vi "Folder Reuse Warning.vi"(8 "error in":errorcluster, 10 "folder names":string[](array[string]), 11 "project ref":refnum<vi>) -> (0 "error out":errorcluster, 3 "proceed?":bool)   [LabVIEW 2021, in "MeasurementClient Editor.lvlib"]
uses:
  MeasurementClient Editor.lvlib
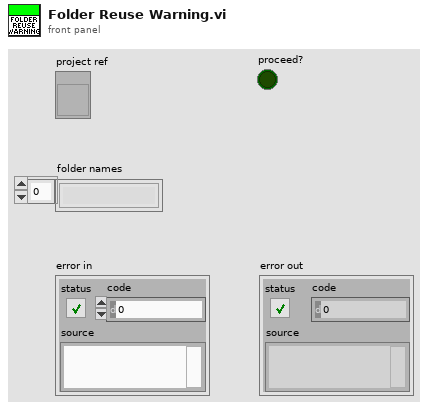
[diagram p1: front panel]
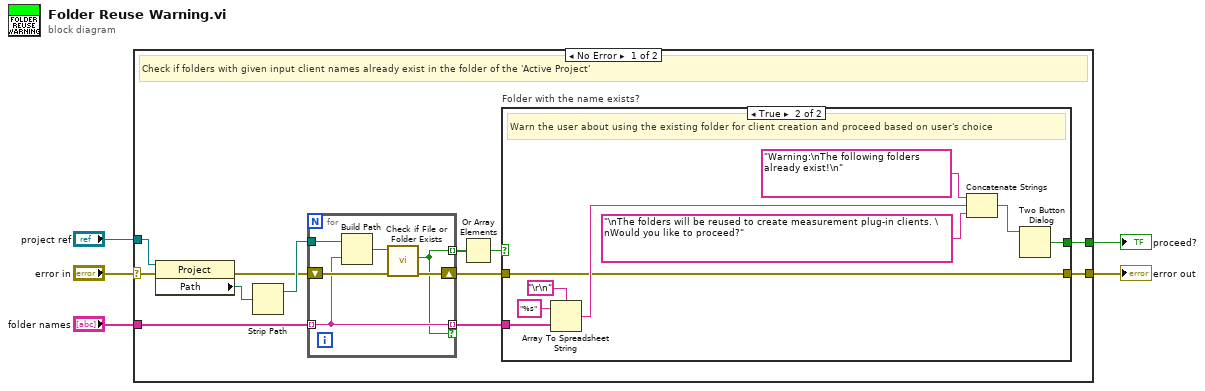
[diagram p0: block diagram]
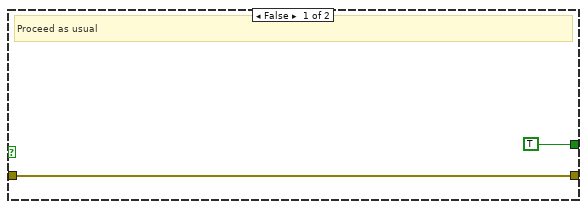
[diagram p2: hidden frame]
diagram:
  n1 = case shown="No Error" "error in" {
    selector: "error in" -> [w17 w35]
    tunnel: [w13 w35] -> w2
    tunnel: "folder names" -> [w12 _]
    tunnel: "project ref" -> [w6 _]
    tunnel: [w9 _] -> w1
    frame No Error {
      # "Check if folders with given input client names already exist in the folder of the 'Active Project'"
      n2 = property class="Project"(reference=w6, error in=w17) -> (error out=w8:errorcluster, "Path"=w16:path)  [unwired: 1 out]
      n3 = Strip Path(path=w16) -> (stripped path=w15:path)  [unwired: 1 out]
      n4 = for {
        tunnel: w15 -> [w34]
        tunnel: w12 -> [w30] mode=indexing
        tunnel: [w29] -> w14 mode=indexing
        tunnel: [w30] -> w11 mode=indexing if=w29
        shift-right: [w31] -> w7
        shift-left: w8 -> [w32]
        n5 = Build Path(base path=w34, name or relative path=w30) -> (appended path=w33:path)
        n6 = call <vilib>:"Check if File or Folder Exists.vi"("error in (no error)"=w32, "path"=w33) -> ("error out"=w31:errorcluster, "file or folder exists?"=w29:bool)  [unwired: 7 in, 1 out]
      }
      n7 = Or Array Elements(Boolean array=w14) -> (logical OR=w10:bool)
      n8 = case "Folder with the name exists?" shown="True" w10 {
        tunnel: [w19 w22] -> w13
        tunnel: w11 -> [_ w28]
        tunnel: [TRUE ("T button?") w24] -> w9
        tunnel: w7 -> [w19 w22]
        frame False {
          # "Proceed as usual"
        }
        frame True {
          # "Warn the user about using the existing folder for client creation and proceed based on user's choice"
          n9 = Array To Spreadsheet String(delimiter (Tab)="\r\n", array=w28, 3:"%s" ("format string")) -> (spreadsheet string=w26:string)
          n10 = Concatenate Strings("Warning:\nThe following folders already exist!\n" ("string"), w26, "\nThe folders will be reused to create measurement plug-in clients. \nWould you like to proceed?" ("string")) -> (w25:string)
          n11 = Two Button Dialog(message=w25) -> (T button?=w24:bool)  [unwired: 2 in]
        }
      }
    }
    frame Error {
      # "Pass"
    }
  }
  "error out" <- w2
  "proceed?" <- w1
